vi "doorlock.vi"() -> (6 "Slide":u8(slide) scale=0.0..100.0)   [LabVIEW 2025]
panel:
  in  "Array":cluster{"Name":string, "Password":string}[](array[cluster])
  in  "Numeric":dbl
  out "name":string
  out "String 2":string
  out "Password":string
  in  "Search Button":bool
  in  "PASSWORD":T1
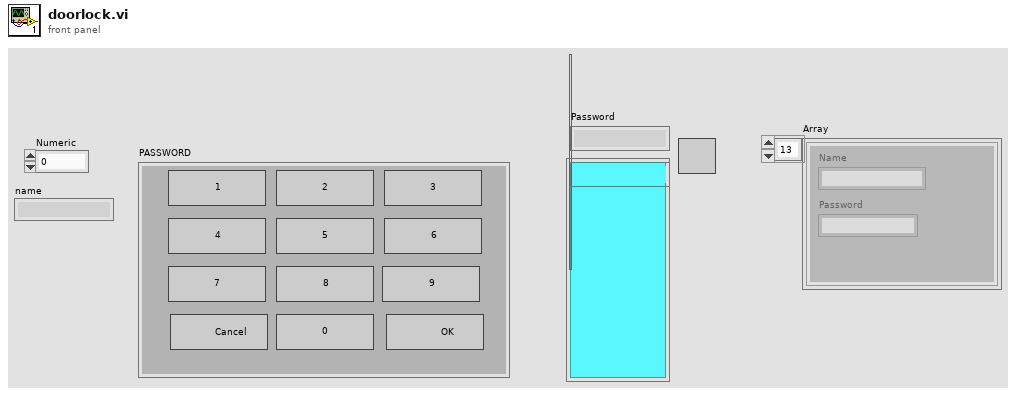
[diagram p1: front panel]
types:
  T1 = cluster{"Blank Button":bool, "Blank Button 2":bool, "Blank Button 3":bool, "Blank Button 4":bool, "Blank Button 5":bool, "Blank Button 6":bool, "Blank Button 7":bool, "Blank Button 8":bool, "Blank Button 9":bool, "Blank Button 10":bool, "OK Button":bool, "Cancel Button":bool}
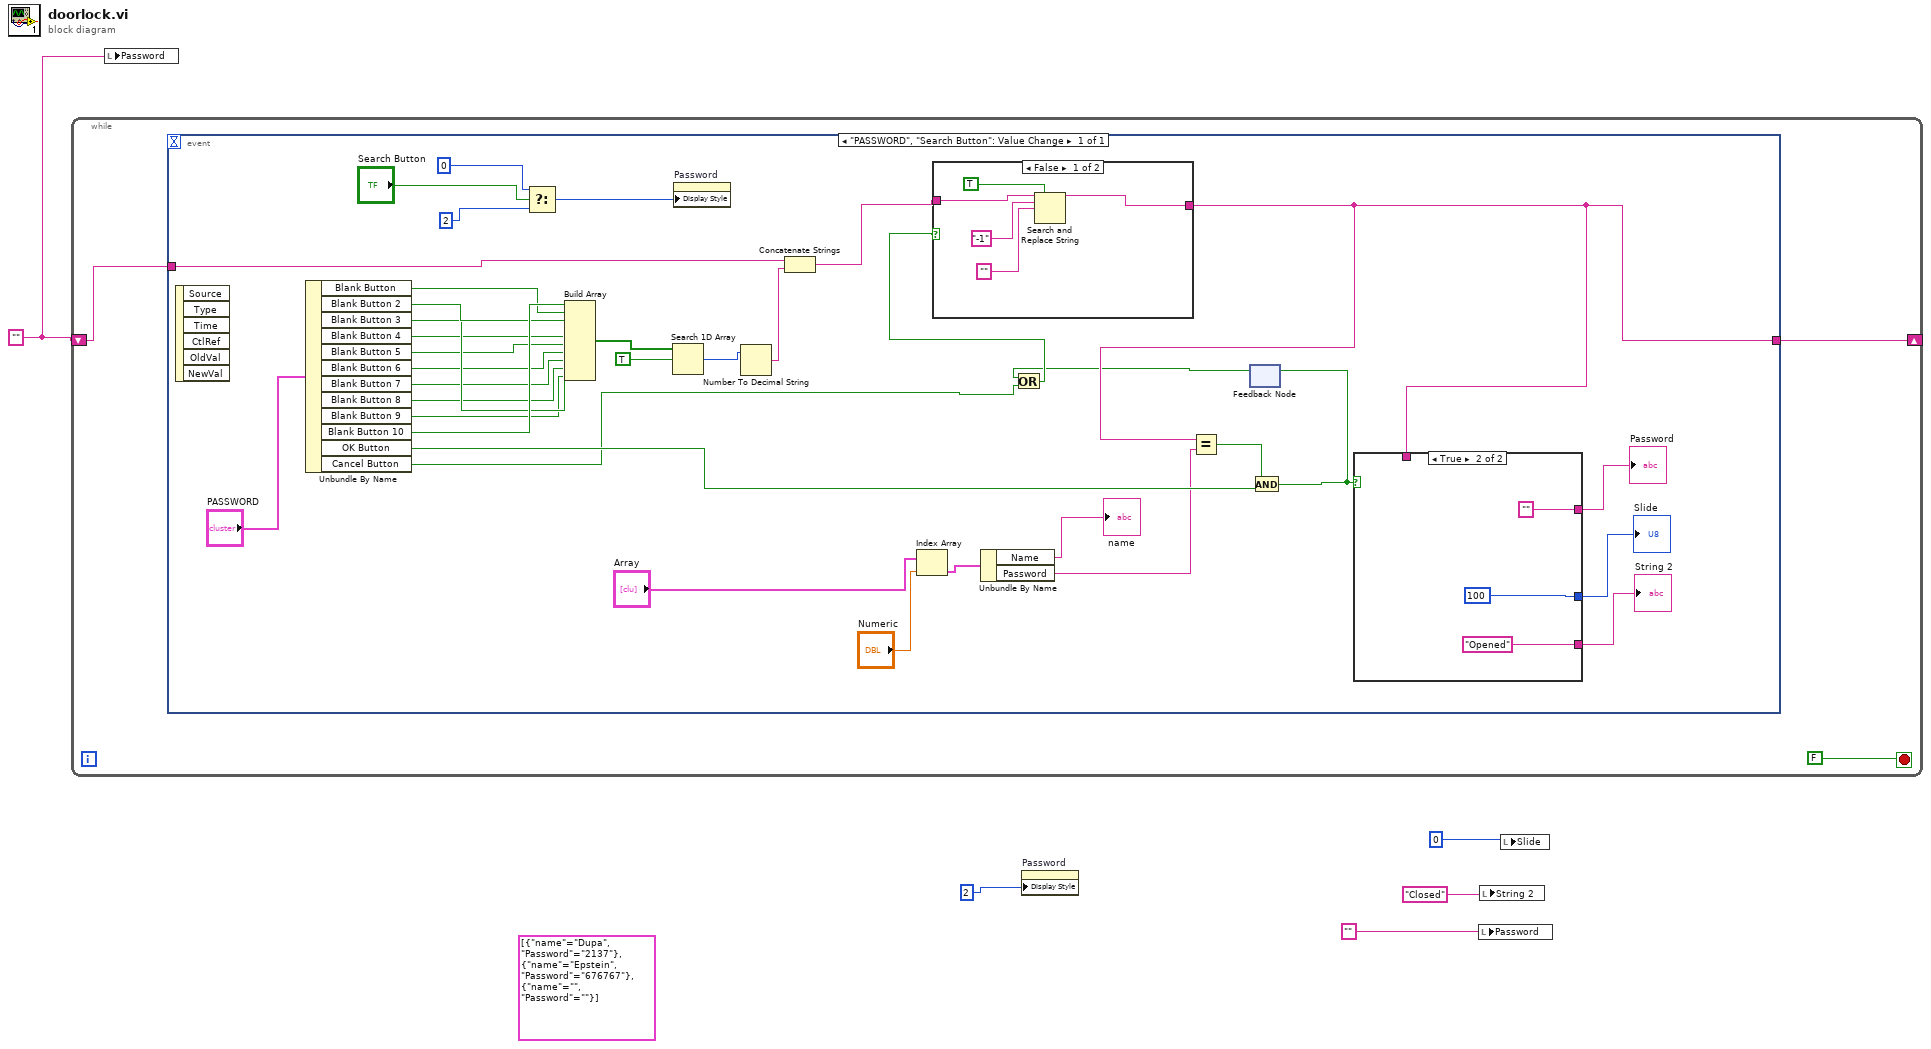
[diagram p0: block diagram]
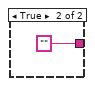
[diagram p2: hidden frame]
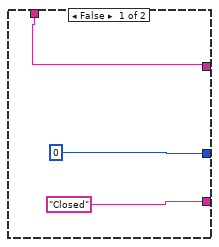
[diagram p3: hidden frame]
diagram:
  (unwired) cluster{"name":string, "Password":string}[] [{"name"="Dupa", "Password"="2137"}, {"name"="Epstein", "Password"="676767"}, {"name"="", "Password"=""}]
  w5 = ""
  n1 = while {
    shift-right: [w7] -> _
    shift-left: w5 -> [w6]
    stop <- FALSE stop-if-true
    n2 = event shown="[0] \"PASSWORD\", \"Search Button\": Value Change" {
      selector: _ -> [_]
      dyn-events: _ -> [_]
      timeout: _ -> [_]
      tunnel: [w22] -> w7
      tunnel: w6 -> [w30]
      event "PASSWORD", "Search Button": Value Change {
        n3 = event-data() -> ()  [unwired: 1 in, 6 out]
        n4 = Unbundle By Name("PASSWORD") -> ("Blank Button"=w39:bool, "Blank Button 2"=w38:bool, "Blank Button 3"=w37:bool, "Blank Button 4"=w36:bool, "Blank Button 5"=w35:bool, "Blank Button 6"=w34:bool, "Blank Button 7"=w33:bool, "Blank Button 8"=w32:bool, "Blank Button 9"=w31:bool, "Blank Button 10"=w40:bool, "OK Button"=w25:bool, "Cancel Button"=w17:bool)
        n5 = Select(t=0, s="Search Button", f=2) -> (s? t:f=w18:i32)
        n6 = Build Array(w40, w39, w38, w37, w36, w35, w34, w33, w32, w31) -> (w43:bool[])
        n7 = Search 1D Array(1D array=w43, element=TRUE) -> (index of element=w41:i32)  [unwired: 1 in]
        n8 = property on="Password" class="Str"("Display Style"=w18) -> ()  [unwired: 2 in, 2 out]
        n9 = Number To Decimal String(number=w41) -> (decimal integer string=w29:string)  [unwired: 1 in]
        n10 = Concatenate Strings(w30, w29) -> (w23:string)
        n11 = Index Array(array="Array", index="Numeric") -> (element=w13:cluster{"Name":string, "Password":string})
        n12 = Unbundle By Name(w13) -> ("Name"=→"name":string, "Password"=w12:string)
        n13 = feedback #1() -> (w15:bool)  [unwired: 1 in]
        n14 = Or(x=w15, y=w17) -> (x .or. y?=w16:bool)
        n15 = case shown="False" w16 {
          tunnel: w23 -> [w49 _]
          tunnel: [w47 ""] -> w22
          frame False {
            n16 = Search and Replace String(replace all?=TRUE ("replace all? (F)"), input string=w49, search string="-1", replace string="" ("replace string (\"\")")) -> (result string=w47:string)  [unwired: 4 in, 3 out]
          }
          frame True {
          }
        }
        n17 = Equal?(x=w22, y=w12) -> (x = y?=w26:bool)
        n18 = And(x=w26, y=w25) -> (x .and. y?=w14:bool)
        n19 = feedback-in #1(w14) -> ()
        n20 = case shown="True" w14 {
          tunnel: [u8 0 ("Slide") u8 100 ("Slide")] -> w28
          tunnel: ["Closed" ("String 2") "Opened" ("String 2")] -> w27
          tunnel: [w51 ""] -> w24
          tunnel: w22 -> [w51 _]
          frame False {
          }
          frame True {
          }
        }
        "Password" <- w24
        "Slide" <- w28
        "String 2" <- w27
      }
    }
  }
  n21 = local write "Password"(w5) -> ()
  n22 = property on="Password" class="Str"("Display Style"=2) -> ()  [unwired: 2 in, 2 out]
  n23 = local write "Password"("" ("Password")) -> ()
  n24 = local write "String 2"("Closed" ("String 2")) -> ()
  n25 = local write "Slide"(u8 0 ("Slide")) -> ()
